vi "Global Message Queue.vi"(6 "Priority?":bool, 7 "Module":T1, 8 "error in (no error)":errorcluster, 9 "Message Data":variant, 10 "State Name":string, 11 "Module Name":string) -> (0 "error out":errorcluster)   [LabVIEW 2019, in "Message Queue.lvlib"]
uses:
  Message Queue.lvlib
  Module Name.ctl
  Shared/TypeDefs/Message Queue Type.ctl
panel:
  in  "timeout in ms (-1)":i32
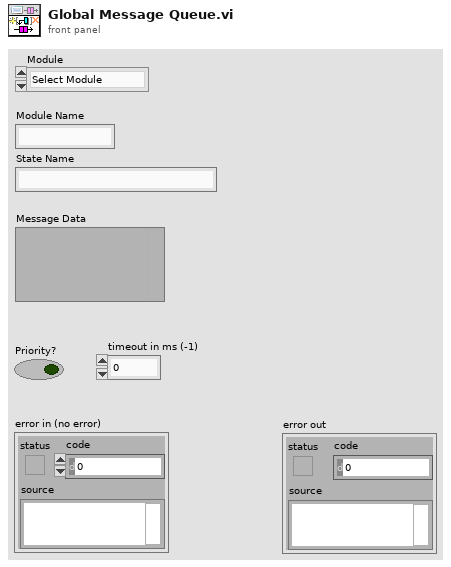
[diagram p1: front panel]
types:
  T1 = typedef "Message Queue.lvlib/Module Name.ctl" = enum16{"Select Module", "Main", "Status"}
  T2 = typedef "Message Queue Type.ctl" = cluster{"Custom State Name":string, "Defined State Name":variant, "Call Chain":string[], "Message Data":variant}
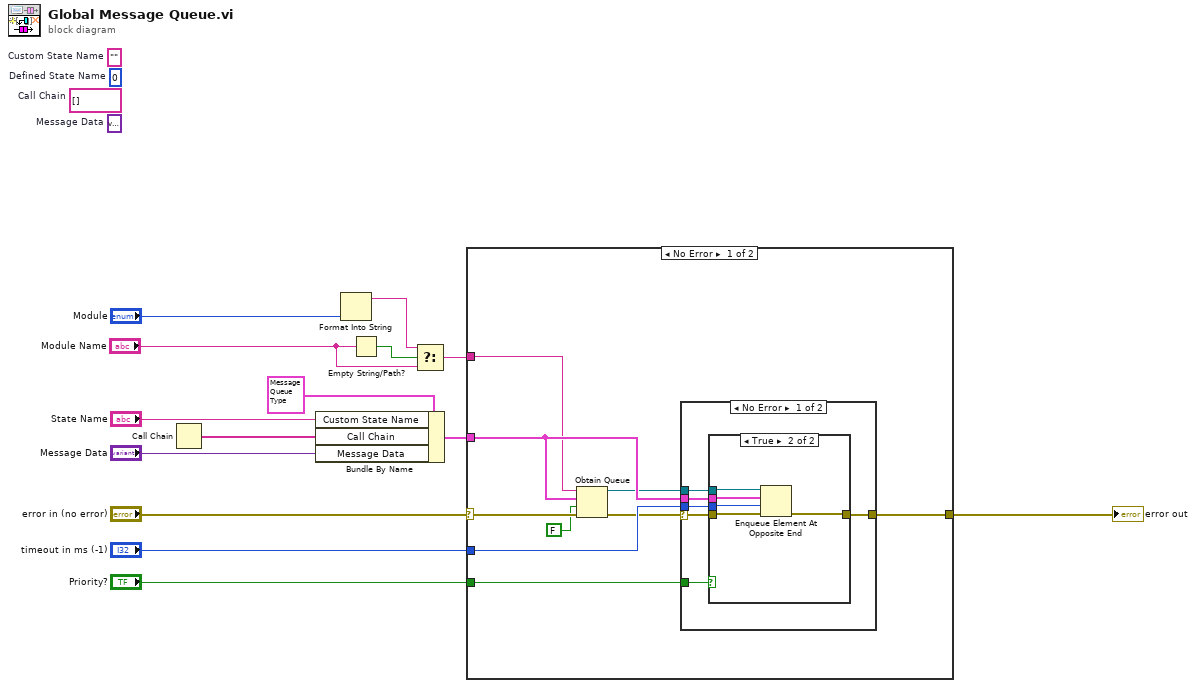
[diagram p0: block diagram]
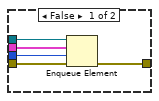
[diagram p2: hidden frame]
diagram:
  (unwired) 0  # Defined State Name
  (unwired) ""  # Custom State Name
  (unwired) variant  # Message Data
  (unwired) string[] []  # Call Chain
  n1 = Call Chain() -> (call chain=w4:string[])
  n2 = Bundle By Name(cluster=T2 {"Custom State Name"="", "Defined State Name"=variant(i32 0), "Call Chain"=[], "Message Data"=variant} ("Message Data"), "Custom State Name"="State Name", "Call Chain"=w4, "Message Data"="Message Data") -> (w2:T2)
  n3 = Format Into String("Module") -> (resulting string=w8:string)  [unwired: 3 in, 1 out]
  n4 = Empty String/Path?(string/path="Module Name") -> (empty?=w9:bool)
  n5 = Select(t=w8, s=w9, f="Module Name") -> (s? t:f=w7:string)
  n6 = case shown="No Error" "error in (no error)" {
    selector: "error in (no error)" -> [w18 w41]
    tunnel: w2 -> [w23 _]
    tunnel: [w22 w41] -> w14
    tunnel: w7 -> [w21 _]
    tunnel: "timeout in ms (-1)" -> [w20 _]
    tunnel: "Priority?" -> [w19 _]
    frame No Error {
      n7 = Obtain Queue(name (unnamed)=w21, element data type=w23, create if not found? (T)=FALSE, error in (no error)=w18) -> (queue out=w17:refnum<queue>, error out=w15:errorcluster)  [unwired: 1 in, 1 out]
      n8 = case shown="No Error" w15 {
        selector: w15 -> [w24 w40]
        tunnel: [w29 w40] -> w22
        tunnel: w17 -> [w28 _]
        tunnel: w23 -> [w27 _]
        tunnel: w20 -> [w26 _]
        tunnel: w19 -> [w25 _]
        frame No Error {
          n9 = case shown="True" w25 {
            tunnel: w24 -> [w34 w36]
            tunnel: [w33 w35] -> w29
            tunnel: w28 -> [w32 w39]
            tunnel: w27 -> [w31 w38]
            tunnel: w26 -> [w30 w37]
            frame False {
              n10 = Enqueue Element(queue=w32, element=w31, timeout in ms (-1)=w30, error in (no error)=w34) -> (error out=w33:errorcluster)  [unwired: 2 out]
            }
            frame True {
              n11 = Enqueue Element At Opposite End(queue=w39, element=w38, timeout in ms (-1)=w37, error in (no error)=w36) -> (error out=w35:errorcluster)  [unwired: 2 out]
            }
          }
        }
        frame Error {
        }
      }
    }
    frame Error {
    }
  }
  "error out" <- w14
